vi "create icon.vi"() -> ()   [LabVIEW 2014]
uses:
  <vilib>/picture/picture.llb/imagedata.ctl
panel:
  out "new picture 2":picture
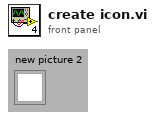
[diagram p1: front panel]
types:
  T1 = typedef "imagedata.ctl" = cluster{"image type":i32, "image depth":i32, "image":u8[], "mask":u8[], "colors":u32[], "Rectangle":cluster{"left":i16, "top":i16, "right":i16, "bottom":i16}}
  T2 = typedef "LVBoundsTypeDef.ctl" = cluster{"Width":u32, "Height":u32}
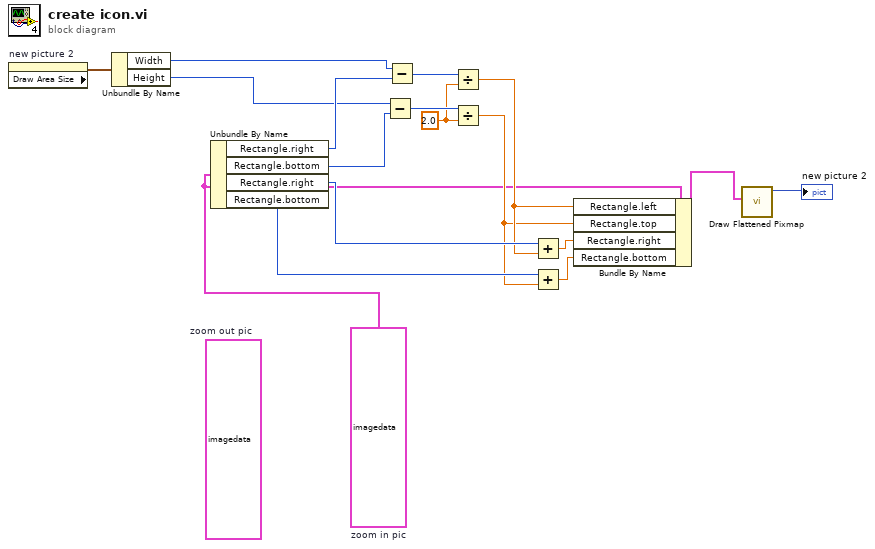
[diagram p0: block diagram]
diagram:
  (unwired) T1 {"image type"=0, "image depth"=24, "image"=[255, 255, 255, 255, 255, 255, 247, 255, 255, 231, 239, 247, 206, 214, 222, 189, 198, 214, 181, 189, 206, 165, 181, 198, 165, 181, 198, 206, 214, 222, 255, 255, 255, 247, 255, 255, 255, 255, 255, 255, 255, 255, 255, 255, 247, 255, 255, 247, 255, 255, 255, 247, 247, 255, 222, 222, 231, 206, 206, 222, 198, 214, 222, 206, 214, 231, 206, 222, 239, 198, 214, 231, 173, 181, 198, 132, 140, 156, 173, 181, 198, 255, 255, 255, 255, 255, 255, 255, 255, 255, 255, 255, 255, 255, 255, 247, 255, 255, 255, 231, 231, 247, 198, 206, 214, 206, 214, 231, 231, 239, 255, 231, 239, 255, 231, 247, 255, 222, 239, 255, 206, 222, 239, 165, 181, 198, 132, 140, 148, 198, 206, 214, 255, 255, 255, 255, 255, 255, 255, 247, 247, 255, 255, 255, 231, 239, 247, 198, 198, 214, 206, 214, 231, 231, 239, 255, 231, 247, 255, 214, 231, 255, 222, 239, 255, 231, 247, 255, 231, 247, 255, 214, 231, 255, 148, 156, 181, 148, 156, 173, 239, 247, 255, 255, 255, 255, 255, 255, 255, 255, 255, 255, 222, 222, 231, 173, 181, 189, 222, 231, 247, 231, 239, 255, 206, 222, 255, 206, 214, 255, 198, 206, 255, 189, 206, 255, 198, 214, 255, 214, 222, 255, 173, 181, 222, 132, 140, 173, 231, 239, 255, 255, 255, 255, 255, 255, 255, 255, 255, 255, 181, 189, 189, 165, 173, 181, 239, 247, 255, 198, 214, 239, 115, 123, 165, 99, 107, 156, 90, 99, 156, 74, 90, 148, 74, 90, 148, 198, 206, 255, 214, 222, 255, 132, 140, 173, 198, 206, 222, 255, 255, 255, 255, 255, 255, 255, 255, 247, 181, 198, 198, 148, 165, 165, 239, 247, 255, 231, 247, 255, 189, 206, 231, 198, 214, 239, 198, 214, 247, 189, 206, 239, 189, 198, 239, 214, 222, 255, 198, 206, 231, 148, 156, 173, 214, 222, 231, 247, 255, 255, 255, 255, 255, 255, 255, 255, 231, 239, 231, 148, 156, 156, 206, 214, 214, 247, 255, 255, 247, 255, 255, 247, 255, 255, 239, 255, 255, 239, 247, 255, 231, 247, 255, 222, 239, 255, 189, 198, 214, 156, 173, 173, 239, 247, 247, 255, 255, 255, 255, 255, 255, 255, 255, 247, 247, 255, 255, 189, 198, 198, 148, 156, 156, 247, 255, 255, 247, 255, 255, 247, 255, 255, 247, 255, 255, 239, 247, 255, 239, 247, 255, 206, 222, 231, 173, 181, 189, 198, 206, 206, 255, 255, 255, 255, 255, 255, 255, 255, 255, 255, 255, 247, 255, 255, 255, 247, 255, 255, 165, 165, 173, 148, 156, 156, 214, 222, 231, 255, 255, 255, 239, 247, 255, 231, 239, 247, 206, 214, 222, 173, 181, 189, 148, 156, 156, 206, 214, 214, 247, 247, 247, 247, 247, 247, 255, 255, 255, 255, 255, 255, 255, 255, 255, 255, 255, 255, 247, 247, 255, 189, 189, 198, 148, 148, 165, 156, 165, 173, 189, 189, 206, 181, 181, 198, 181, 181, 198, 189, 198, 206, 173, 173, 181, 123, 123, 132, 123, 123, 123, 247, 247, 255, 255, 255, 255, 255, 255, 255, 255, 255, 255, 255, 255, 255, 255, 255, 255, 255, 255, 255, 231, 231, 239, 222, 222, 231, 206, 214, 222, 214, 222, 231, 239, 239, 247, 255, 255, 255, 222, 222, 239, 140, 140, 148, 82, 82, 82, 115, 107, 115, 247, 239, 247, 255, 255, 255, 255, 255, 255, 255, 255, 255, 255, 255, 255, 255, 255, 255, 255, 255, 255, 255, 255, 255, 255, 255, 255, 255, 255, 255, 255, 255, 255, 255, 255, 255, 255, 255, 255, 206, 206, 206, 148, 148, 148, 82, 82, 82, 132, 123, 132, 231, 231, 239, 255, 255, 255, 255, 255, 255, 255, 255, 255, 247, 247, 247, 255, 255, 255, 255, 255, 255, 255, 255, 255, 255, 255, 255, 255, 255, 247, 255, 255, 255, 255, 255, 247, 255, 255, 255, 198, 198, 198, 148, 148, 148, 82, 74, 82, 156, 156, 156, 255, 255, 255, 255, 255, 255, 255, 255, 255, 255, 255, 255, 255, 255, 255, 255, 255, 255, 255, 255, 255, 255, 255, 255, 255, 255, 255, 255, 255, 255, 255, 255, 255, 255, 255, 255, 255, 255, 255, 206, 206, 206, 148, 148, 148, 214, 222, 214, 255, 255, 255, 255, 255, 247, 255, 255, 255, 255, 255, 255, 255, 255, 255, 255, 255, 255, 255, 255, 255, 255, 255, 255, 255, 255, 255, 255, 255, 255, 255, 255, 255, 255, 255, 255, 255, 255, 255, 255, 255, 255, 255, 255, 247, 255, 255, 255], "mask"=[], "colors"=[], "Rectangle"={"left"=0, "top"=0, "right"=16, "bottom"=16}}  # zoom out pic
  w1 = T1 {"image type"=0, "image depth"=24, "image"=[255, 255, 247, 255, 255, 247, 247, 255, 255, 231, 239, 239, 206, 214, 222, 181, 198, 214, 181, 189, 206, 165, 189, 198, 165, 181, 189, 198, 214, 214, 247, 255, 255, 247, 255, 247, 255, 255, 255, 255, 255, 255, 255, 247, 255, 255, 255, 255, 255, 255, 255, 247, 255, 247, 214, 222, 231, 189, 198, 214, 198, 206, 222, 214, 231, 255, 198, 214, 239, 189, 214, 231, 173, 189, 206, 123, 140, 148, 173, 181, 189, 255, 255, 255, 255, 255, 255, 255, 255, 255, 255, 255, 255, 255, 255, 255, 247, 255, 255, 231, 239, 239, 189, 198, 214, 214, 222, 247, 231, 239, 255, 222, 239, 255, 206, 222, 255, 222, 239, 255, 206, 222, 255, 165, 181, 206, 123, 140, 156, 198, 206, 214, 255, 255, 255, 255, 255, 255, 255, 247, 255, 255, 255, 255, 247, 247, 255, 189, 198, 206, 206, 214, 239, 231, 239, 255, 231, 239, 255, 189, 206, 255, 115, 132, 181, 198, 214, 255, 231, 247, 255, 214, 231, 255, 140, 156, 181, 148, 156, 173, 239, 247, 255, 255, 255, 255, 255, 255, 255, 255, 255, 255, 222, 231, 239, 173, 181, 198, 222, 231, 255, 222, 231, 255, 206, 222, 255, 165, 181, 239, 90, 107, 165, 181, 198, 255, 198, 214, 255, 206, 222, 255, 165, 181, 214, 132, 140, 165, 231, 239, 247, 247, 255, 255, 255, 255, 255, 255, 255, 255, 198, 198, 206, 173, 173, 189, 239, 247, 255, 198, 206, 247, 115, 123, 173, 99, 115, 173, 82, 99, 156, 66, 90, 148, 74, 90, 148, 189, 214, 255, 206, 222, 255, 132, 140, 165, 198, 206, 222, 255, 255, 255, 255, 255, 255, 255, 255, 255, 206, 206, 214, 156, 156, 173, 231, 239, 255, 231, 239, 255, 198, 214, 255, 156, 173, 214, 66, 82, 132, 165, 189, 231, 181, 206, 247, 206, 231, 255, 189, 206, 231, 148, 156, 173, 214, 222, 222, 255, 255, 255, 255, 255, 255, 255, 255, 255, 239, 239, 239, 148, 148, 156, 214, 214, 231, 247, 255, 255, 247, 255, 255, 198, 214, 239, 82, 99, 132, 198, 222, 255, 231, 247, 255, 214, 239, 255, 181, 198, 214, 156, 173, 181, 239, 247, 255, 255, 255, 255, 255, 255, 255, 255, 255, 247, 255, 255, 255, 189, 189, 198, 148, 156, 165, 239, 247, 255, 247, 255, 255, 231, 247, 255, 189, 206, 231, 231, 247, 255, 231, 247, 255, 206, 222, 231, 173, 181, 189, 198, 206, 214, 247, 255, 255, 255, 255, 255, 255, 255, 255, 255, 255, 255, 255, 255, 255, 239, 239, 239, 165, 173, 173, 148, 148, 156, 206, 222, 222, 247, 255, 255, 231, 247, 255, 231, 247, 255, 206, 214, 222, 173, 181, 189, 140, 156, 156, 206, 214, 214, 247, 247, 247, 247, 247, 247, 255, 255, 255, 255, 255, 255, 255, 255, 255, 255, 255, 255, 247, 247, 255, 181, 189, 189, 148, 156, 156, 156, 165, 165, 181, 189, 198, 173, 189, 189, 181, 189, 189, 189, 198, 206, 165, 173, 181, 123, 123, 132, 123, 123, 123, 247, 247, 255, 255, 255, 255, 255, 255, 255, 255, 255, 255, 255, 255, 255, 255, 255, 255, 255, 255, 255, 231, 231, 231, 214, 222, 214, 214, 214, 214, 214, 214, 222, 239, 239, 247, 255, 255, 255, 222, 222, 231, 148, 140, 148, 82, 82, 90, 115, 107, 115, 247, 239, 247, 255, 255, 255, 255, 255, 255, 255, 255, 255, 255, 255, 255, 255, 255, 255, 255, 255, 255, 255, 255, 255, 255, 255, 255, 255, 255, 255, 255, 255, 255, 255, 255, 255, 255, 255, 255, 206, 206, 214, 148, 148, 156, 82, 82, 90, 132, 123, 132, 231, 231, 239, 255, 255, 255, 255, 255, 255, 255, 255, 255, 255, 255, 255, 247, 247, 247, 255, 255, 255, 255, 255, 255, 255, 255, 255, 255, 255, 255, 255, 255, 255, 255, 255, 255, 255, 255, 255, 198, 198, 206, 148, 148, 148, 74, 74, 74, 156, 156, 156, 255, 255, 255, 255, 255, 255, 255, 255, 255, 255, 255, 255, 255, 255, 255, 255, 255, 255, 255, 255, 255, 255, 255, 255, 255, 255, 255, 255, 255, 255, 255, 255, 255, 255, 255, 255, 255, 255, 255, 206, 206, 206, 148, 148, 140, 214, 222, 206, 255, 255, 255, 255, 255, 255, 255, 255, 255, 255, 255, 255, 255, 255, 255, 255, 255, 255, 255, 255, 255, 255, 255, 255, 255, 255, 255, 255, 255, 255, 255, 255, 255, 255, 255, 255, 255, 255, 255, 255, 255, 255, 247, 255, 239, 255, 255, 247], "mask"=[], "colors"=[], "Rectangle"={"left"=0, "top"=0, "right"=16, "bottom"=16}}  # zoom in pic
  w10 = 2.0 ("y")
  n1 = property on="new picture 2" class="Pict"() -> ("Draw Area Size"=w17:T2)  [unwired: 2 in, 2 out]
  n2 = Unbundle By Name(w17) -> ("Width"=w16:u32, "Height"=w14:u32)
  n3 = Unbundle By Name(w1) -> ("Rectangle.right"=w15:i16, "Rectangle.bottom"=w12:i16, "Rectangle.right"=w9:i16, "Rectangle.bottom"=w6:i16)
  n4 = Subtract(x=w14, y=w12) -> (x-y=w11:u32)
  n5 = Subtract(x=w16, y=w15) -> (x-y=w13:u32)
  n6 = Divide(x=w13, y=w10) -> (x/y=w8:dbl)
  n7 = Divide(x=w11, y=w10) -> (x/y=w5:dbl)
  n8 = Add(x=w9, y=w8) -> (x+y=w7:dbl)
  n9 = Add(x=w6, y=w5) -> (x+y=w4:dbl)
  n10 = Bundle By Name(cluster=w1, "Rectangle.left"=w8, "Rectangle.top"=w5, "Rectangle.right"=w7, "Rectangle.bottom"=w4) -> (w2:T1)
  n11 = call <vilib>:"Draw Flattened Pixmap.vi"("image data"=w2) -> ("new picture"=→"new picture 2":picture)  [unwired: 8 in]
